vi "WebErrorMsgProcess.vi"(0 "WebErrorMsg":string) -> ()   [LabVIEW 2011]
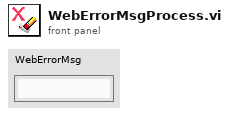
[diagram p1: front panel]
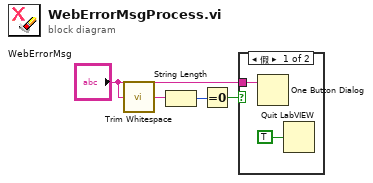
[diagram p0: block diagram]
diagram:
  n1 = call <vilib>:"Trim Whitespace.vi"("string"="WebErrorMsg") -> ("trimmed string"=w4:string)  [unwired: 1 in]
  n2 = String Length(string=w4) -> (length=w3:i32)
  n3 = Equal To 0?(x=w3) -> (x = 0?=w2:bool)
  n4 = case shown="假" w2 {
    tunnel: "WebErrorMsg" -> [w6 _]
    frame False {
      n5 = One Button Dialog(message=w6) -> ()  [unwired: 1 in, 1 out]
      n6 = Quit LabVIEW(quit? (T)=TRUE ("退出？(T)")) -> ()
    }
    frame True {
    }
  }
